vi "RunningAnts.vi"(8 "error in (no error)":errorcluster, 11 "Ants in":refnum<class "Ants.lvclass">) -> (0 "error out":errorcluster, 3 "Ants out":refnum<class "Ants.lvclass">)   [LabVIEW 2021, in "Ants.lvclass"]
uses:
  <resource>/plugins/NIIconEditor/Class/Ants/Ants.lvclass
  <vilib>/picture/picture.llb/imagedata.ctl
panel:
  in  "image data":T1
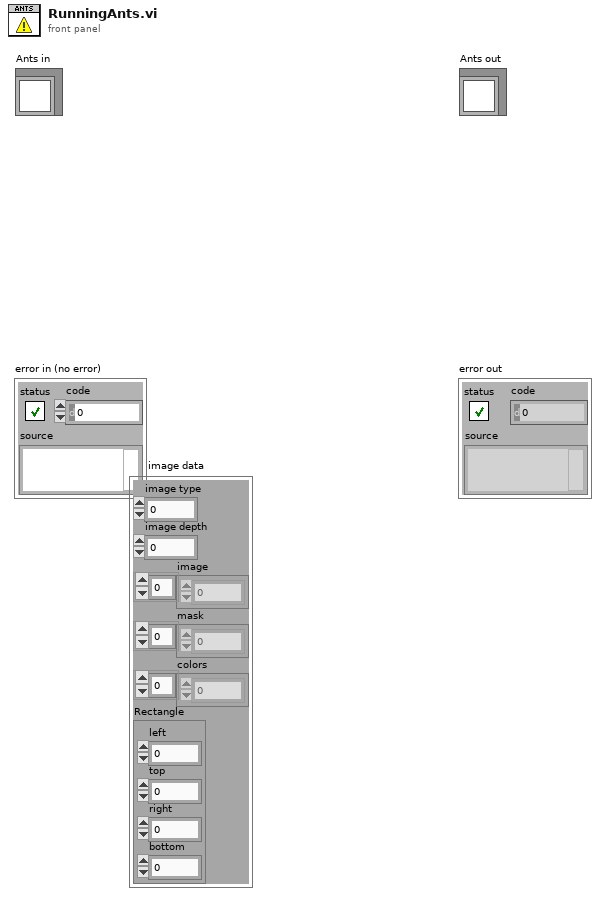
[diagram p1: front panel]
types:
  T1 = typedef "imagedata.ctl" = cluster{"image type":i32, "image depth":i32, "image":u8[], "mask":u8[], "colors":u32[], "Rectangle":cluster{"left":i16, "top":i16, "right":i16, "bottom":i16}}
  T2 = cluster{"Left":i32, "Bottom":i32, "Right":i32, "Bottom":i32}[]
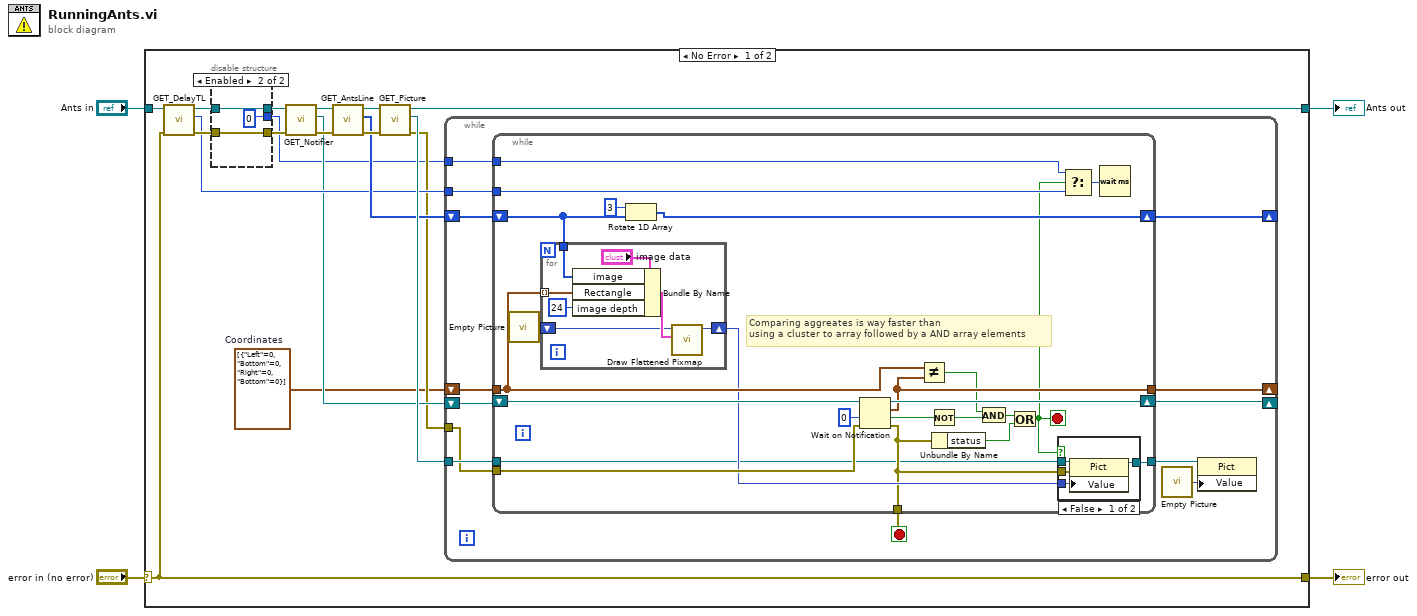
[diagram p0: block diagram]
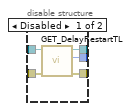
[diagram p2: hidden frame]
diagram:
  n1 = case shown="No Error" "error in (no error)" {
    selector: "error in (no error)" -> [w9 w80]
    tunnel: [w9 w80] -> w3
    tunnel: [w21 w79] -> w1
    tunnel: "Ants in" -> [w22 w79]
    frame No Error {
      w6 = T2 [{"Left"=0, "Bottom"=0, "Right"=0, "Bottom"=0}]  # Coordinates
      n2 = call-dynamic "GET_DelayTL.vi"("error in (no error)"=w9, "Ants.lvclass in"=w22) -> ("error out"=w20:errorcluster, "Delay TL (ms)"=w10:u32, "Ants.lvclass out"=w16:refnum<class "Ants.lvclass">)  [unwired: 7 out]
      n3 = disable-structure shown="Enabled" {
        disable-tunnel: w20 -> [w27 w28]
        disable-tunnel: [w26 w28] -> w19
        disable-tunnel: w16 -> [w25 w29]
        disable-tunnel: [w24 w29] -> w15
        disable-tunnel: [w23 u32 0 ("Delay Restart TL (ms)")] -> w5
        frame Disabled {
          n4 = call-dynamic "GET_DelayRestartTL.vi"("error in (no error)"=w27, "Ants.lvclass in"=w25) -> ("error out"=w26:errorcluster, "Delay Restart TL (ms)"=w23:u32, "Ants.lvclass out"=w24:refnum<class "Ants.lvclass">)  [unwired: 7 out]
        }
        frame Enabled {
        }
      }
      n5 = call-dynamic "GET_Notifier.vi"("error in (no error)"=w19, "Ants.lvclass in"=w15) -> ("error out"=w18:errorcluster, "Notifier"=w8:refnum<notifier>, "Ants.lvclass out"=w14:refnum<class "Ants.lvclass">)  [unwired: 7 out]
      n6 = call-dynamic "GET_AntsLine.vi"("error in (no error)"=w18, "Ants.lvclass in"=w14) -> ("error out"=w17:errorcluster, "Ants Line"=w11:u8[], "Ants.lvclass out"=w13:refnum<class "Ants.lvclass">)  [unwired: 7 out]
      n7 = call-dynamic "GET_Picture.vi"("error in (no error)"=w17, "Ants.lvclass in"=w13) -> ("error out"=w7:errorcluster, "Picture"=w12:refnum<vi>, "Ants.lvclass out"=w21:refnum<class "Ants.lvclass">)  [unwired: 7 out]
      n8 = while {
        shift-right: [w42] -> _
        shift-left: w11 -> [w43]
        tunnel: w12 -> [w41]
        tunnel: w10 -> [w38]
        shift-right: [w35] -> _
        shift-left: w8 -> [w36]
        tunnel: w7 -> [w37]
        shift-right: [w33] -> _
        shift-left: w6 -> [w32]
        tunnel: w5 -> [w31]
        stop <- w34 stop-if-true
        n9 = while {
          shift-right: [w65] -> w42
          shift-left: w43 -> [w63]
          tunnel: w41 -> [w45]
          tunnel: [w44] -> w40
          tunnel: w37 -> [w49]
          tunnel: w38 -> [w51]
          shift-right: [w62] -> w35
          shift-left: w36 -> [w61]
          tunnel: [w47] -> w34
          tunnel: [w57] -> w33
          tunnel: w32 -> [w58]
          tunnel: w31 -> [w50]
          stop <- w46 stop-if-true
          # "Comparing aggreates is way faster than\nusing a cluster to array followed by a AND array elements"
          n10 = call "Empty Picture"() -> ("empty picture"=w64:picture)
          n11 = for {
            shift-right: [w76] -> w48
            shift-left: w64 -> [w75]
            tunnel: w63 -> [w74]
            tunnel: w58 -> [w72] mode=indexing
            n12 = Bundle By Name(cluster="image data", "image"=w74, "Rectangle"=w72, "image depth"=24) -> (w78:T1)
            n13 = call <vilib>:"Draw Flattened Pixmap.vi"("image data"=w78, "picture"=w75) -> ("new picture"=w76:picture)  [unwired: 7 out]
          }
          n14 = Rotate 1D Array(1:w63, 2:3 ("n")) -> (0:w65:u8[])
          n15 = Wait on Notification(notifier=w61, timeout in ms (-1)=0, error in (no error)=w49) -> (notifier out=w62:refnum<notifier>, notification=w57:T2, timed out?=w60:bool, error out=w47:errorcluster)  [unwired: 1 out]
          n16 = Not Equal?(x=w58, y=w57) -> (x != y?=w54:bool)
          n17 = Not(x=w60) -> (.not. x?=w59:bool)
          n18 = Unbundle By Name(w47) -> ("status"=w55:bool)
          n19 = And(x=w54, y=w59) -> (x .and. y?=w56:bool)
          n20 = Or(x=w56, y=w55) -> (x .or. y?=w46:bool)
          n21 = case shown="False" w46 {
            tunnel: w48 -> [w70 _]
            tunnel: w47 -> [w69 _]
            tunnel: w45 -> [w68 w71]
            tunnel: [w67 w71] -> w44
            frame False {
              n22 = property class="Pict"(reference=w68, error in=w69, "Value"=w70) -> (reference out=w67:refnum<vi>)  [unwired: 1 out]
            }
            frame True {
            }
          }
          n23 = Select(t=w50, s=w46, f=w51) -> (s? t:f=w52:u32)
          n24 = Wait (ms)(milliseconds to wait=w52) -> ()  [unwired: 1 out]
        }
        n25 = call "Empty Picture"() -> ("empty picture"=w39:picture)
        n26 = property class="Pict"(reference=w40, "Value"=w39) -> ()  [unwired: 1 in, 2 out]
      }
    }
    frame Error {
    }
  }
  "error out" <- w3
  "Ants out" <- w1
